vi "Display.vi"(8 "error in":errorcluster, 11 "Input (I32) in":refnum<class "Input (I32).lvclass">) -> (0 "error out":errorcluster, 3 "Input (I32) out":refnum<class "Input (I32).lvclass">)   [LabVIEW 2021, in "Pop-Up.lvlib" / "Input (I32).lvclass"]
doc: "This vi will display the input pop up waiting for a type I32 input from the user\n\n<b>Code Developed By:</b> +\nDaniel Coons +\nhttps://github.com/danielcoons/tsc-pop-up"
uses:
  Input (I32).lvclass
  C:/Development/Open Source/tsc-pop-up/Popup/Popup.lvclass
  Input (I32).lvclass/Input (I32).ctl
  Popup/Popup.lvclass/Popup.ctl
  Popup/Data Member Access/Read Theme.vi
  Theme/Theme.lvclass
  Popup/Popup.lvclass
  user32.dll
panel:
  out "header":bool
  out "2D Picture":picture
  in  "OK Button":bool
  in  "Input":i32
  out "String":string
  out "Input value out":i32=1 min=1
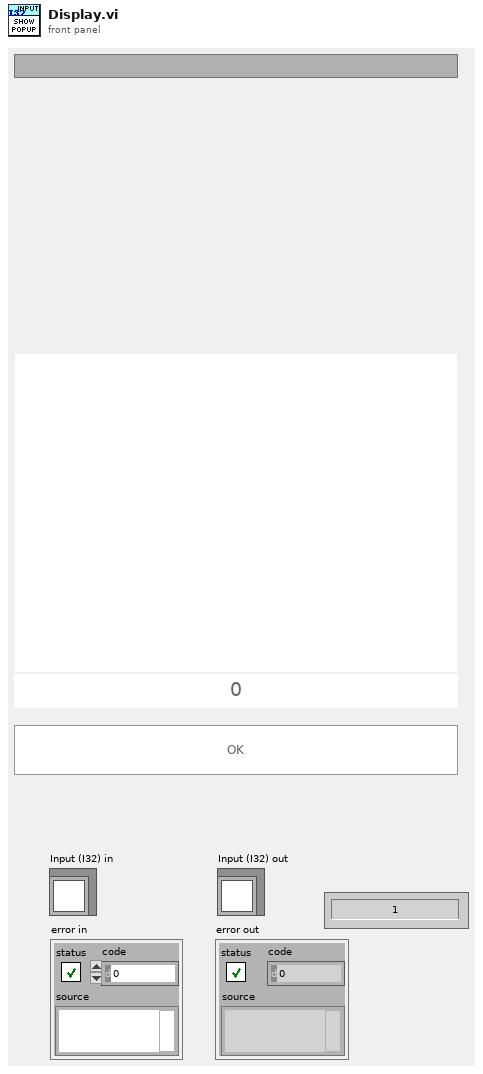
[diagram p1: front panel]
types:
  T1 = typedef "LVPoint32TypeDef.ctl" = cluster{"Horizontal":i32, "Vertical":i32}
  T2 = typedef "LVPositionTypeDef.ctl" = cluster{"Left":i32, "Top":i32}
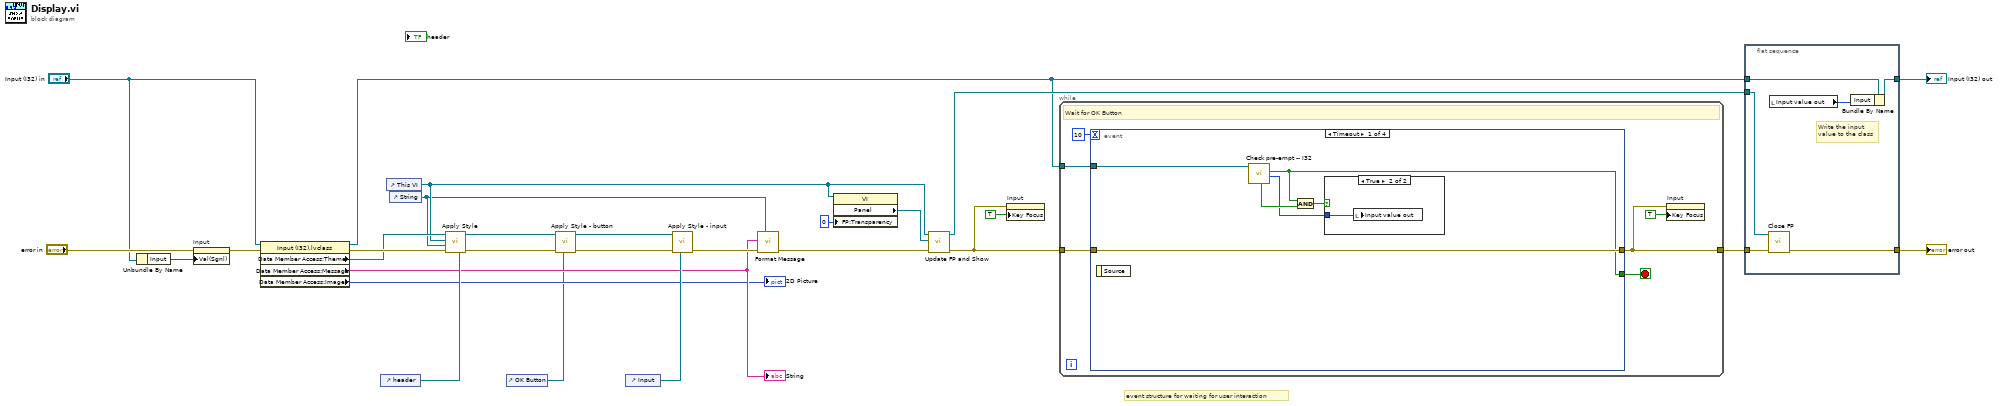
[diagram p0: block diagram]
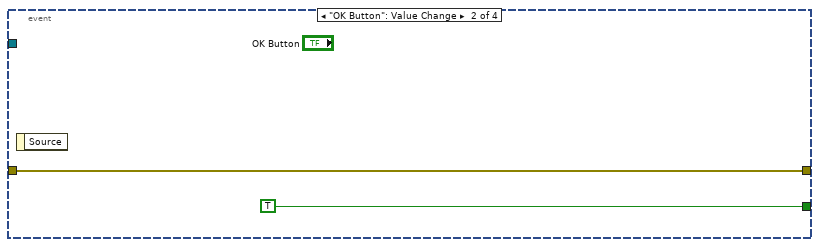
[diagram p3: hidden frame]
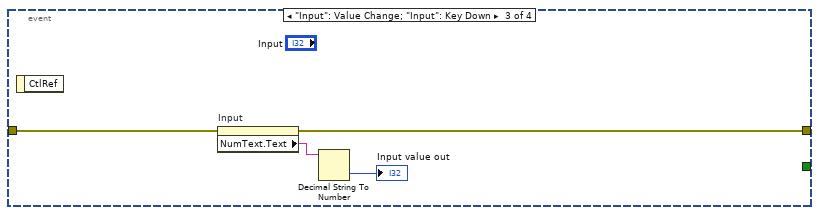
[diagram p4: hidden frame]
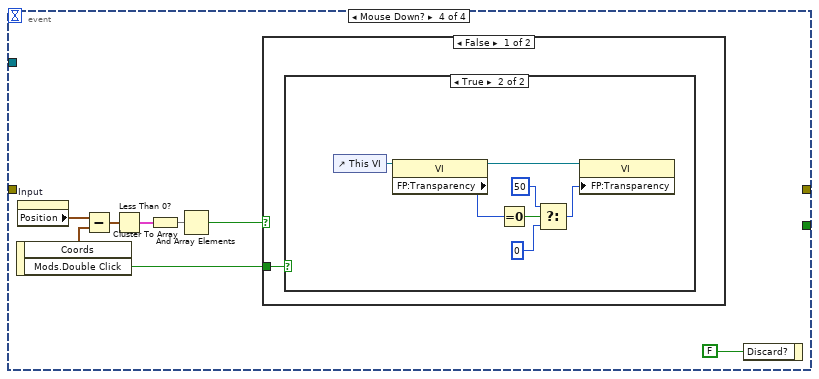
[diagram p5: hidden frame]
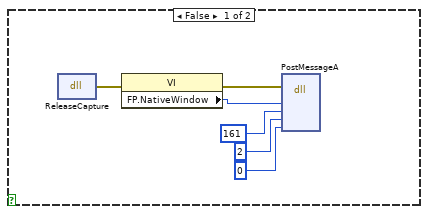
[diagram p6: hidden frame]
diagram:
  # "event structure for waiting for user interaction"
  n1 = Unbundle By Name("Input (I32) in") -> ("Input"=w24:i32)
  n2 = property on="Input" class="DigNum (strict)"(error in="error in", "Val(Sgnl)"=w24) -> (error out=w10:errorcluster)  [unwired: 1 in, 1 out]
  n3 = property class="Input (I32).lvclass"(reference="Input (I32) in", error in=w10) -> (reference out=w1:refnum<class "Input (I32).lvclass">, error out=w20:errorcluster, "Data Member Access:Theme"=w18:refnum<class "Theme.lvclass">, "Data Member Access:Message"=w6:string, "Data Member Access:Image"=→"2D Picture":picture)
  "String" <- w6
  n4 = control-ref of="header"() -> (w16:refnum<vi>)
  n5 = control-ref of="This VI"() -> (w17:refnum<vi>)
  n6 = control-ref of="String"() -> (w5:refnum<vi>)
  n7 = call "Apply Style.vi"("header ref"=w16, "error in"=w20, "message ref"=w5, "pop up ref"=w17, "Theme in"=w18) -> ("error out"=w19:errorcluster, "Theme out"=w14:refnum<class "Theme.lvclass">)  [unwired: 5 in]
  n8 = control-ref of="OK Button"() -> (w3:refnum<vi>)
  n9 = call "Apply Style - button.vi"("button ref"=w3, "error in"=w19, "Theme in"=w14) -> ("error out"=w15:errorcluster, "Theme out"=w12:refnum<class "Theme.lvclass">)  [unwired: 7 in]
  n10 = control-ref of="Input"() -> (w11:refnum<vi>)
  n11 = call "Apply Style - input.vi"("input ref"=w11, "error in (no error)"=w15, "Theme in"=w12) -> ("error out"=w13:errorcluster)  [unwired: 7 in, 1 out]
  n12 = call "Format Message.vi"("formatted string"=w5, "error in"=w13, "String Input"=w6) -> ("error out"=w21:errorcluster)  [unwired: 7 in, 1 out]
  n13 = property class="VI"(reference=w17, "FP:Transparency"=u8 0 ("Front Panel Window:Transparency")) -> ("Panel"=w22:refnum<vi>)  [unwired: 1 in, 2 out]
  n14 = call "Update FP and Show.vi"("error in (no error)"=w21, "Panel Ref"=w22, "VI in"=w17) -> ("error out"=w8:errorcluster, "VI out"=w7:refnum<vi>)  [unwired: 7 in]
  n15 = property on="Input" class="DigNum (strict)"(error in=w8, "Key Focus"=TRUE) -> ()  [unwired: 1 in, 2 out]
  n16 = while {
    tunnel: w8 -> [w34]
    tunnel: [w29] -> w25
    tunnel: w1 -> [w32]
    stop <- w33 stop-if-true
    # "Wait for OK Button"
    n17 = event shown="[0] Timeout" {
      selector: _ -> [_ _ _ _]
      dyn-events: _ -> [_ _ _ _]
      timeout: 10 -> [_ _ _ _]
      tunnel: w34 -> [w40 w43 w47 _]
      tunnel: [w40 w43 w45 _] -> w29
      tunnel: [w35 TRUE _ _] -> w33
      tunnel: w32 -> [w36 _ _ _]
      event Timeout {
        n18 = event-data() -> ()  [unwired: 1 in, 1 out]
        n19 = call "Check pre-empt -- I32.vi"("_Popup in"=w36) -> ("Value?"=w37:i32, "Pre-empted?"=w35:bool, "Type Match?"=w39:bool)  [unwired: 7 in, 1 out]
        n20 = Compound Arithmetic op=AND(w35, w39) -> (w38:bool)
        n21 = case shown="True" w38 {
          tunnel: w37 -> [_ w41]
          frame False {
          }
          frame True {
            n22 = local write "Input value out"(w41) -> ()
          }
        }
      }
      event "OK Button": Value Change {
        n23 = event-data() -> ()  [unwired: 1 in, 1 out]
      }
      event "Input": Value Change; "Input": Key Down {
        n24 = event-data() -> ()  [unwired: 1 in, 1 out]
        n25 = property on="Input" class="DigNum (strict)"(error in=w47) -> (error out=w45:errorcluster, "NumText.Text"=w46:string)  [unwired: 1 in, 1 out]
        n26 = Decimal String To Number(string=w46) -> (number=→"Input value out":i32)  [unwired: 2 in, 1 out]
      }
      event Mouse Down? {
        n27 = event-data() -> ("Coords"=w50:T1, "Mods.Double Click"=w48:bool)  [unwired: 1 in]
        n28 = property on="Input" class="DigNum (strict)"() -> ("Position"=w54:T2)  [unwired: 2 in, 2 out]
        n29 = Subtract(x=w54, y=w50) -> (x-y=w53:T2)
        n30 = Less Than 0?(x=w53) -> (x < 0?=w52:cluster{"Left":bool, "Top":bool})
        n31 = Cluster To Array(cluster=w52) -> (array=w51:bool[])
        n32 = And Array Elements(Boolean array=w51) -> (logical AND=w49:bool)
        n33 = case shown="False" w49 {
          tunnel: w48 -> [w56 _]
          frame False {
            n34 = case shown="True" w56 {
              frame False {
                n35 = dll-call lib="user32.dll" fn="ReleaseCapture"() -> (error out=w60:errorcluster)  [unwired: 4 in, 1 out]
                n36 = property class="VI"(error in=w60) -> (error out=w61:errorcluster, "FP.NativeWindow"=w62:u64)  [unwired: 1 in, 1 out]
                n37 = dll-call lib="user32.dll" fn="PostMessageA"(error in=w61, "hWnd"=w62, "Msg"=161, "wParam"=2, "lParam"=0) -> ()  [unwired: 7 in, 2 out]
              }
              frame True {
                n38 = control-ref of="This VI"() -> (w69:refnum<vi>)
                n39 = property class="VI"(reference=w69) -> (reference out=w67:refnum<vi>, "FP:Transparency"=w68:u8)  [unwired: 1 in, 1 out]
                n40 = Equal To 0?(x=w68) -> (x = 0?=w66:bool)
                n41 = Select(t=u8 50, s=w66, f=u8 0) -> (s? t:f=w65:u8)
                n42 = property class="VI"(reference=w67, "FP:Transparency"=w65) -> ()  [unwired: 1 in, 2 out]
              }
            }
          }
          frame True {
          }
        }
        n43 = event-data("Discard?"=FALSE) -> ()  [unwired: 1 in, 1 out]
      }
    }
    n44 = property on="Input" class="DigNum (strict)"(error in=w29, "Key Focus"=TRUE) -> ()  [unwired: 1 in, 2 out]
  }
  n45 = flat-sequence {
    tunnel: w25 -> [w75]
    tunnel: [w71] -> w27
    tunnel: w1 -> [w74]
    tunnel: [w73] -> w26
    tunnel: w7 -> [w70]
    frame #0 {
      # "Write the input\nvalue to the class"
      n46 = call "Close FP.vi"("error in (no error)"=w75, "VI in"=w70) -> ("error out"=w71:errorcluster)  [unwired: 9 in]
      n47 = local read "Input value out"() -> (w72:i32)
      n48 = Bundle By Name(cluster=w74, "Input"=w72) -> (w73:refnum<class "Input (I32).lvclass">)
    }
  }
  "error out" <- w27
  "Input (I32) out" <- w26
